vi "All_ThingsSummer2020.vi"() -> ()   [LabVIEW 2020]
uses:
  Examples/_Subs/OpenDiagram/Open_XControl.xctl
  Subs/RestAPI.ctl
  Subs/ColorText/ColorGlobals.vi
  Subs/SystemLink/SL_Subs/SystemLink_Write_String.vi
  Subs/JSON_Formats.vi
panel:
  in  "OpenDiag":refnum<vi>(xcontrol)
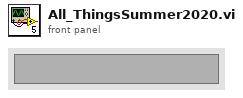
[diagram p1: front panel]
types:
  T1 = typedef "RestAPI.ctl" = cluster{"headers 2":string, "headers":string, "body":string}
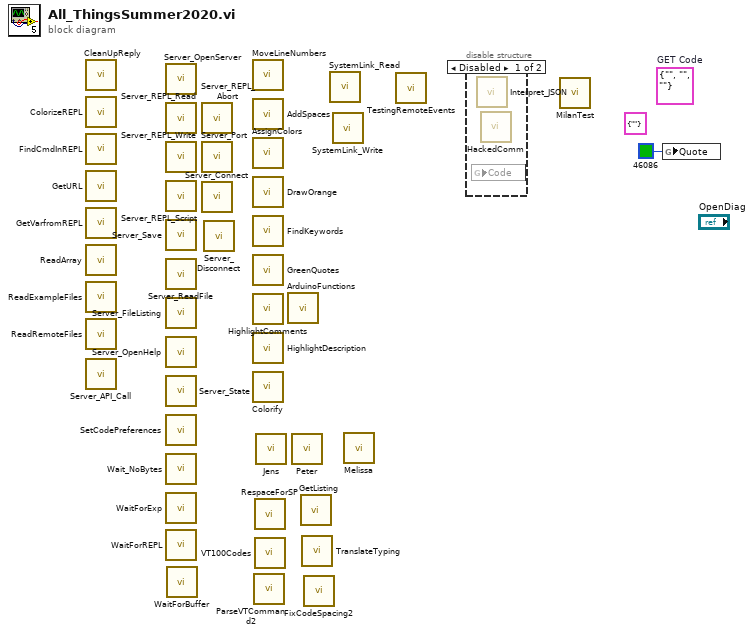
[diagram p0: block diagram]
diagram:
  (unwired) cluster{"Code":string} {"Code"=""} ("Code")
  (unwired) T1 {"headers 2"="", "headers"="", "body"=""}  # GET Code
  n1 = call "CleanUpReply.vi"() -> ()  [unwired: 11 in, 1 out]
  n2 = call "ColorizeREPL.vi"() -> ()  [unwired: 10 in, 1 out]
  n3 = call "FindCmdInREPL.vi"() -> ()  [unwired: 11 in, 1 out]
  n4 = call "GetURL.vi"() -> ()  [unwired: 8 in, 4 out]
  n5 = call "GetVarfromREPL.vi"() -> ()  [unwired: 10 in, 2 out]
  n6 = call "ReadArray.vi"() -> ()  [unwired: 11 in, 1 out]
  n7 = call "ReadExampleFiles.vi"() -> ()  [unwired: 12 in]
  n8 = call "ReadRemoteFiles.vi"() -> ()  [unwired: 12 in]
  n9 = call "Server_API_Call.vi"() -> ()  [unwired: 9 in, 3 out]
  n10 = call "Server_OpenServer.vi"() -> ()  [unwired: 11 in, 1 out]
  n11 = call "Server_REPL_Read.vi"() -> ()  [unwired: 9 in, 3 out]
  n12 = call "Server_REPL_Write.vi"() -> ()  [unwired: 11 in, 1 out]
  n13 = call "Server_REPL_Script.vi"() -> ()  [unwired: 11 in, 1 out]
  n14 = call "Server_Save.vi"() -> ()  [unwired: 11 in, 1 out]
  n15 = call "Server_ReadFile.vi"() -> ()  [unwired: 10 in, 2 out]
  n16 = call "Server_FileListing.vi"() -> ()  [unwired: 8 in, 4 out]
  n17 = call "Server_OpenHelp.vi"() -> ()  [unwired: 11 in, 1 out]
  n18 = call "Server_State.vi"() -> ()  [unwired: 9 in, 3 out]
  n19 = call "SetCodePreferences.vi"() -> ()  [unwired: 12 in]
  n20 = call "Wait_NoBytes.vi"() -> ()  [unwired: 10 in, 2 out]
  n21 = call "WaitForExp.vi"() -> ()  [unwired: 10 in, 2 out]
  n22 = call "WaitForREPL.vi"() -> ()  [unwired: 10 in, 2 out]
  n23 = call "WaitForBuffer.vi"() -> ()  [unwired: 10 in, 2 out]
  n24 = call "Server_REPL_Abort.vi"() -> ()  [unwired: 11 in, 1 out]
  n25 = call "Server_Port.vi"() -> ()  [unwired: 11 in, 1 out]
  n26 = call "Server_Connect.vi"() -> ()  [unwired: 11 in, 1 out]
  n27 = call "Server_Disconnect.vi"() -> ()  [unwired: 11 in, 1 out]
  n28 = call "MoveLineNumbers.vi"() -> ()  [unwired: 12 in]
  n29 = call "AddSpaces.vi"() -> ()  [unwired: 10 in, 2 out]
  n30 = call "AssignColors.vi"() -> ()  [unwired: 11 in, 1 out]
  n31 = call "DrawOrange.vi"() -> ()  [unwired: 11 in, 1 out]
  n32 = call "FindKeywords.vi"() -> ()  [unwired: 11 in, 1 out]
  n33 = call "GreenQuotes.vi"() -> ()  [unwired: 11 in, 1 out]
  n34 = call "HighlightComments.vi"() -> ()  [unwired: 11 in, 1 out]
  n35 = call "HighlightDescription.vi"() -> ()  [unwired: 11 in, 1 out]
  n36 = call "Colorify.vi"() -> ()  [unwired: 12 in]
  n37 = call "ParseVTCommand2.vi"() -> ()  [unwired: 7 in, 5 out]
  n38 = call "RespaceForSP.vi"() -> ()  [unwired: 11 in, 1 out]
  n39 = call "VT100Codes.vi"() -> ()  [unwired: 11 in, 1 out]
  n40 = call "Jens.vi"() -> ()  [unwired: 12 in]
  n41 = call "ArduinoFunctions.vi"() -> ()  [unwired: 11 in, 1 out]
  n42 = call "Peter.vi"() -> ()  [unwired: 12 in]
  n43 = call "GetListing.vi"() -> ()  [unwired: 9 in, 3 out]
  n44 = call "TranslateTyping.vi"() -> ()  [unwired: 11 in, 1 out]
  n45 = call "FixCodeSpacing2.vi"() -> ()  [unwired: 11 in, 1 out]
  n46 = call "SystemLink_Read.vi"() -> ()  [unwired: 8 in, 4 out]
  n47 = call-poly "SystemLink_Write.vi"() -> ()  [unwired: 11 in, 1 out]
  n48 = call "Melissa.vi"() -> ()  [unwired: 12 in]
  n49 = call "TestingRemoteEvents.vi"() -> ()  [unwired: 12 in]
  n50 = disable-structure shown="Disabled" {
    frame Disabled {
      n51 = global read "JSON_Formats.vi" "Code"() -> ()  [unwired: 1 in]
      n52 = call "Interpret_JSON.vi"() -> ()  [unwired: 9 in, 3 out]
      n53 = call "HackedComm.vi"() -> ()  [unwired: 10 in, 2 out]
    }
    frame Enabled {
    }
  }
  n54 = call "MilanTest.vi"() -> ()  [unwired: 12 in]
  n55 = global write "ColorGlobals.vi" "Quote"(u32 46086 ("Quote")) -> ()
